vi "Read Panel.vi"(11 "Panel Actor in":refnum<class "Panel Actor.lvclass">) -> (2 "Panel":refnum<class "Panel.lvclass">)   [LabVIEW 2017, in "MGI-Panel Actor.lvlib" / "Panel Actor.lvclass"]
doc: "Reads the panel for the actor.\n\nWarning: The panel can change at any time, so you should not store this object.\nWarning: Calling any methods on the Panel object may cause errors in the framework. Typically this VI should only be used when initializing a new Panel class that will be launched as a nested Panel.\n\n----\nCopyright: MGI 2018\nAuthor: Derek Trepanier"
uses:
  Panel Actor.lvclass
  panel-manager/Source/Panel/Panel.lvclass
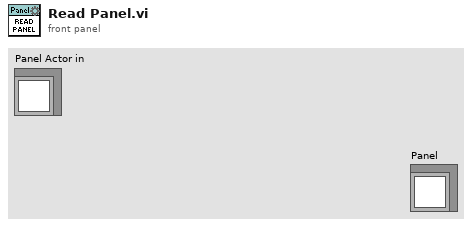
[diagram p1: front panel]
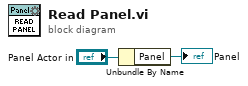
[diagram p0: block diagram]
diagram:
  n1 = Unbundle By Name("Panel Actor in") -> ("Panel"=→"Panel":refnum<class "Panel.lvclass">)
